vi "Main Processing Loop.vi"(0 "InteractionProcessor in":refnum<class "InteractionProcessor.lvclass">, 5 "Internal Message Queue":refnum<queue>, 7 "Notification Message Queue":refnum<queue>, 9 "Wait Time":u32 caption="ms" step=1, 11 "error in (no error)":errorcluster, 12 "Results Notifier":refnum<notifier>) -> (4 "InteractionProcessor out":refnum<class "InteractionProcessor.lvclass">, 15 "error out":errorcluster)   [LabVIEW 2023, in "HAF.lvlib" / "InteractionProcessor.lvclass"]
doc: "Waits for messages to appear on the queue and then processes it. In many respects it resembles a state machine in that each processed message adds another to the queue so that processing will continue in the next iteration.\n\nIt is responsible for actually processing all Command Directors in sequence once it receives the Process message to do so."
uses:
  InteractionProcessor.lvclass
  ReadCommand/ReadCommand.lvclass
  Message.ctl
  HAF.lvlib
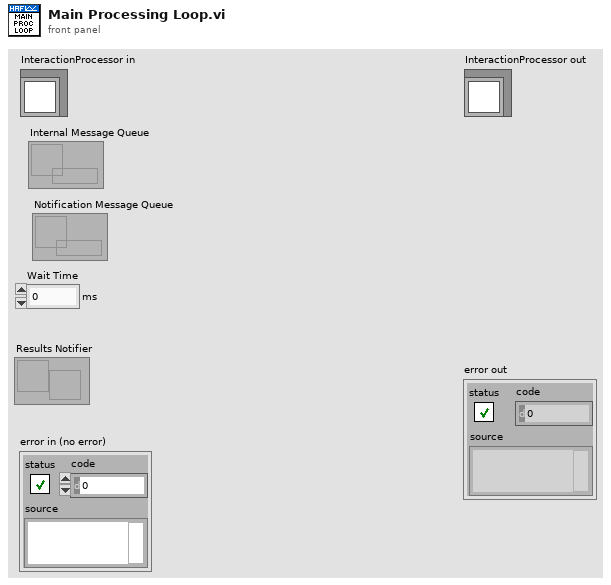
[diagram p1: front panel]
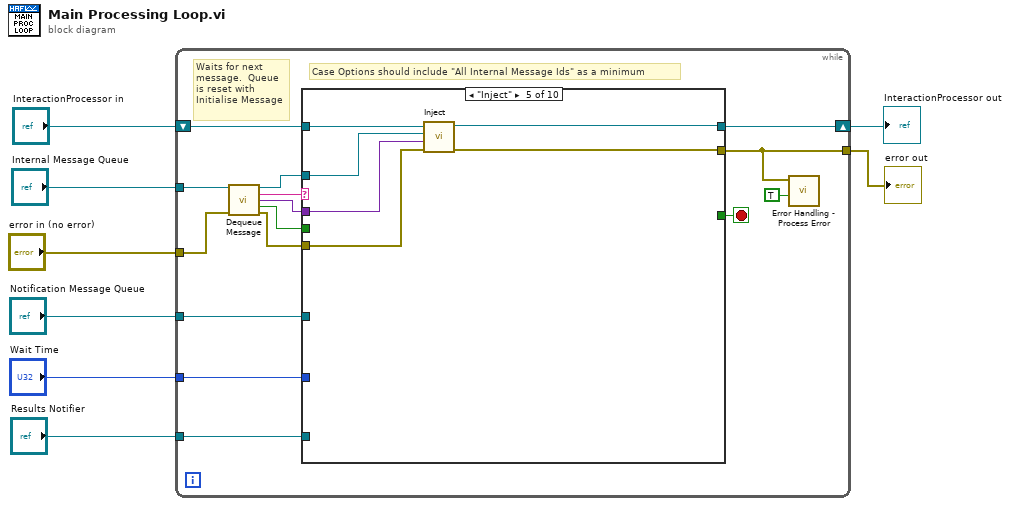
[diagram p0: block diagram]
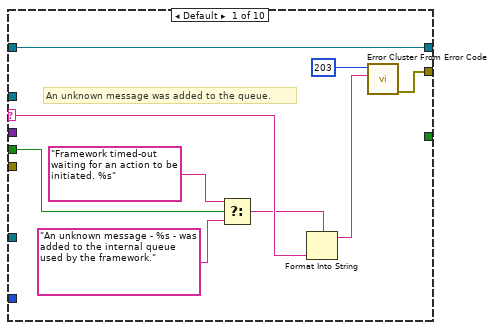
[diagram p2: hidden frame]
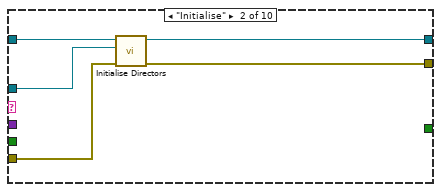
[diagram p3: hidden frame]
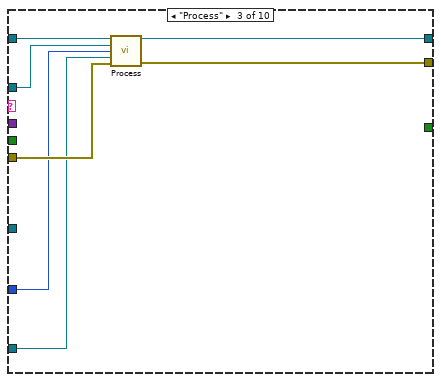
[diagram p4: hidden frame]
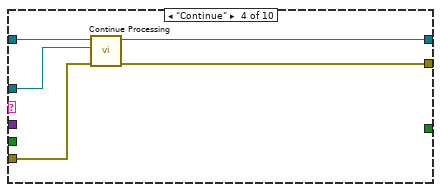
[diagram p5: hidden frame]
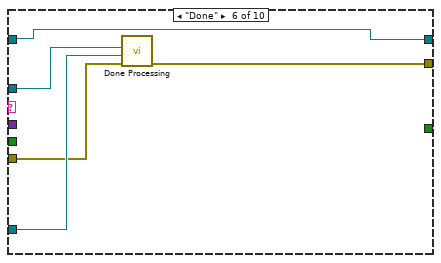
[diagram p6: hidden frame]
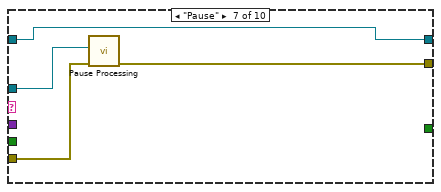
[diagram p7: hidden frame]
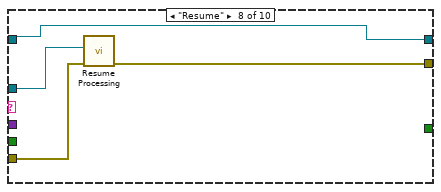
[diagram p8: hidden frame]
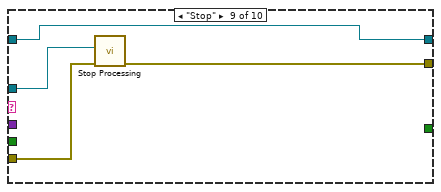
[diagram p9: hidden frame]
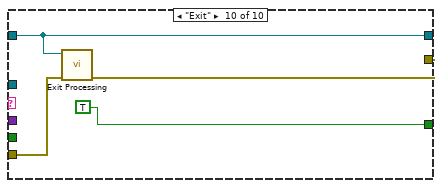
[diagram p10: hidden frame]
diagram:
  n1 = while {
    tunnel: "Internal Message Queue" -> [w23]
    tunnel: "error in (no error)" -> [w22]
    tunnel: "Notification Message Queue" -> [w15]
    shift-right: [w11] -> w2
    shift-left: "InteractionProcessor in" -> [w16]
    tunnel: "Wait Time" -> [w13]
    tunnel: "Results Notifier" -> [w12]
    tunnel: [w10] -> w1
    stop <- w14 stop-if-true
    # "Waits for next\nmessage.  Queue\nis reset with \nInitialise Message"
    # "Case Options should include \"All Internal Message Ids\" as a minimum"
    n2 = call "Dequeue Message.vi"("Message Queue In"=w23, "error in (no error)"=w22) -> ("Message Queue Out"=w21:refnum<queue>, "Message Id"=w20:string, "Message Data"=w19:variant, "Timed Out"=w18:bool, "error out"=w17:errorcluster)  [unwired: 9 in]
    n3 = case shown="\"Inject\"" w20 {
      selector: w20 -> [w29 _ _ _ _ _ _ _ _ _]
      tunnel: w21 -> [_ w36 w43 w46 w54 w58 w62 w68 w70 _]
      tunnel: w19 -> [_ _ _ _ w53 _ _ _ _ _]
      tunnel: w18 -> [w32 _ _ _ _ _ _ _ _ _]
      tunnel: w17 -> [_ w37 w42 w48 w52 w59 w64 w67 w72 w76]
      tunnel: [w26 w35 w40 w45 w50 w57 w63 w66 w71 w75] -> w10
      tunnel: [w25 w33 w41 w47 w51 w56 w61 w65 w69 w74] -> w11
      tunnel: w16 -> [w25 w34 w44 w49 w55 w56 w61 w65 w69 w74]
      tunnel: w15 -> [_ _ _ _ _ w60 _ _ _ _]
      tunnel: [_ _ _ _ _ _ _ _ _ TRUE] -> w14
      tunnel: w13 -> [_ _ w39 _ _ _ _ _ _ _]
      tunnel: w12 -> [_ _ w38 _ _ _ _ _ _ _]
      frame Default {
        # "An unknown message was added to the queue."
        n4 = Select(t="Framework timed-out waiting for an action to be initiated. %s", s=w32, f="An unknown message - %s - was added to the internal queue used by the framework.") -> (s? t:f=w24:string)
        n5 = Format Into String(format string=w24, w29) -> (resulting string=w28:string)  [unwired: 2 in, 1 out]
        n6 = call <vilib>:"Error Cluster From Error Code.vi"("error message (\"\")"=w28, "error code (0)"=203) -> ("error out"=w26:errorcluster)  [unwired: 7 in]
      }
      frame "Initialise" {
        n7 = call "Initialise Directors.vi"("error in (no error)"=w37, "Internal Message Queue"=w36, "InteractionProcessor in"=w34) -> ("error out"=w35:errorcluster, "InteractionProcessor out"=w33:refnum<class "InteractionProcessor.lvclass">)  [unwired: 7 in]
      }
      frame "Process" {
        n8 = call "Process.vi"("InteractionProcessor in"=w44, "Internal Message Queue"=w43, "Wait Time"=w39, "Results Notifier"=w38, "error in (no error)"=w42) -> ("InteractionProcessor out"=w41:refnum<class "InteractionProcessor.lvclass">, "error out"=w40:errorcluster)  [unwired: 9 in]
      }
      frame "Continue" {
        n9 = call "Continue Processing.vi"("error in (no error)"=w48, "Internal Message Queue"=w46, "InteractionProcessor in"=w49) -> ("error out"=w45:errorcluster, "InteractionProcessor out"=w47:refnum<class "InteractionProcessor.lvclass">)  [unwired: 7 in]
      }
      frame "Inject" {
        n10 = call "Inject.vi"("error in (no error)"=w52, "Injection Data"=w53, "Internal Message Queue"=w54, "InteractionProcessor in"=w55) -> ("error out"=w50:errorcluster, "InteractionProcessor out"=w51:refnum<class "InteractionProcessor.lvclass">)  [unwired: 6 in]
      }
      frame "Done" {
        n11 = call "Done Processing.vi"("error in (no error)"=w59, "Notification Message Queue"=w60, "Internal Message Queue"=w58) -> ("error out"=w57:errorcluster)  [unwired: 8 in]
      }
      frame "Pause" {
        n12 = call "Pause Processing.vi"("error in (no error)"=w64, "Internal Message Queue"=w62) -> ("error out"=w63:errorcluster)  [unwired: 9 in]
      }
      frame "Resume" {
        n13 = call "Resume Processing.vi"("error in (no error)"=w67, "Queue in"=w68) -> ("error out"=w66:errorcluster)  [unwired: 9 in]
      }
      frame "Stop" {
        n14 = call "Stop Processing.vi"("error in (no error)"=w72, "Queue in"=w70) -> ("error out"=w71:errorcluster)  [unwired: 9 in]
      }
      frame "Exit" {
        n15 = call "Exit Processing.vi"("error in (no error)"=w76, "InteractionProcessor in"=w74) -> ("error out"=w75:errorcluster)  [unwired: 9 in]
      }
    }
    n16 = call "Error Handling - Process Error.vi"("Exit on Error"=TRUE, "error to process"=w10) -> ()  [unwired: 9 in, 1 out]
  }
  "error out" <- w1
  "InteractionProcessor out" <- w2
